vi "Process.vi"(0 "reference in":refnum<class "SSH.lvclass">, 5 "error in":errorcluster) -> (14 "reference out":refnum<class "SSH.lvclass">, 19 "error out":errorcluster)   [LabVIEW 2023, in "HPS-17000-PowerModule.lvlib" / "SSH.lvclass"]
uses:
  SSH.lvclass
  <vilib>/Utility/SystemLogging/NI_SystemLogging.lvlib
panel:
  out "error info":errorcluster
  out "Last Command":string
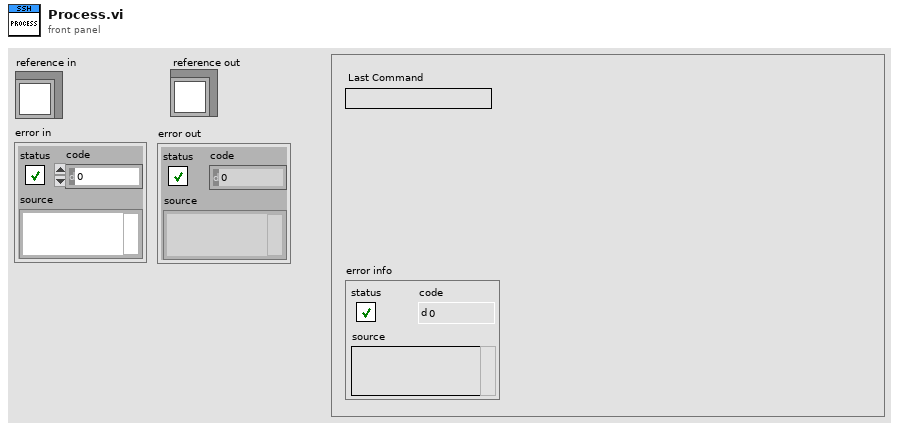
[diagram p1: front panel]
types:
  T1 = cluster{"Core":cluster{"Timeout":i32, "Events":cluster{"EventsToProcess":refnum<event-registration>}, "EventFromProcess":refnum<user-event>, "ProcessSyncQueue":refnum<queue>, "QueueFromProcess":refnum<queue>, "Command":string, "Data":variant}, "Process ID":i32, "Script Prefix":string, "Log File":string, "Full Command":string, "Script Name":string, "Standard Input":string, "Console Listbox":refnum<vi>, "Script Complete Event":refnum<user-event>}
  T2 = enum32{"Invalid", "Standard", "Closed", "Hidden", "Minimized", "Maximized"}
  T3 = cluster{"EventsToProcess":refnum<event-registration>}
  T4 = typedef "HPS-17000-PowerModule.lvlib/SSH.lvclass/ObjectAttributes.ctl" = cluster{"Update Rate (ms)":i32, "Console Listbox":refnum<vi>, "Full Command":string, "Script Name":string, "Log File":string, "IP Address":string, "Script Complete Event":refnum<user-event>}
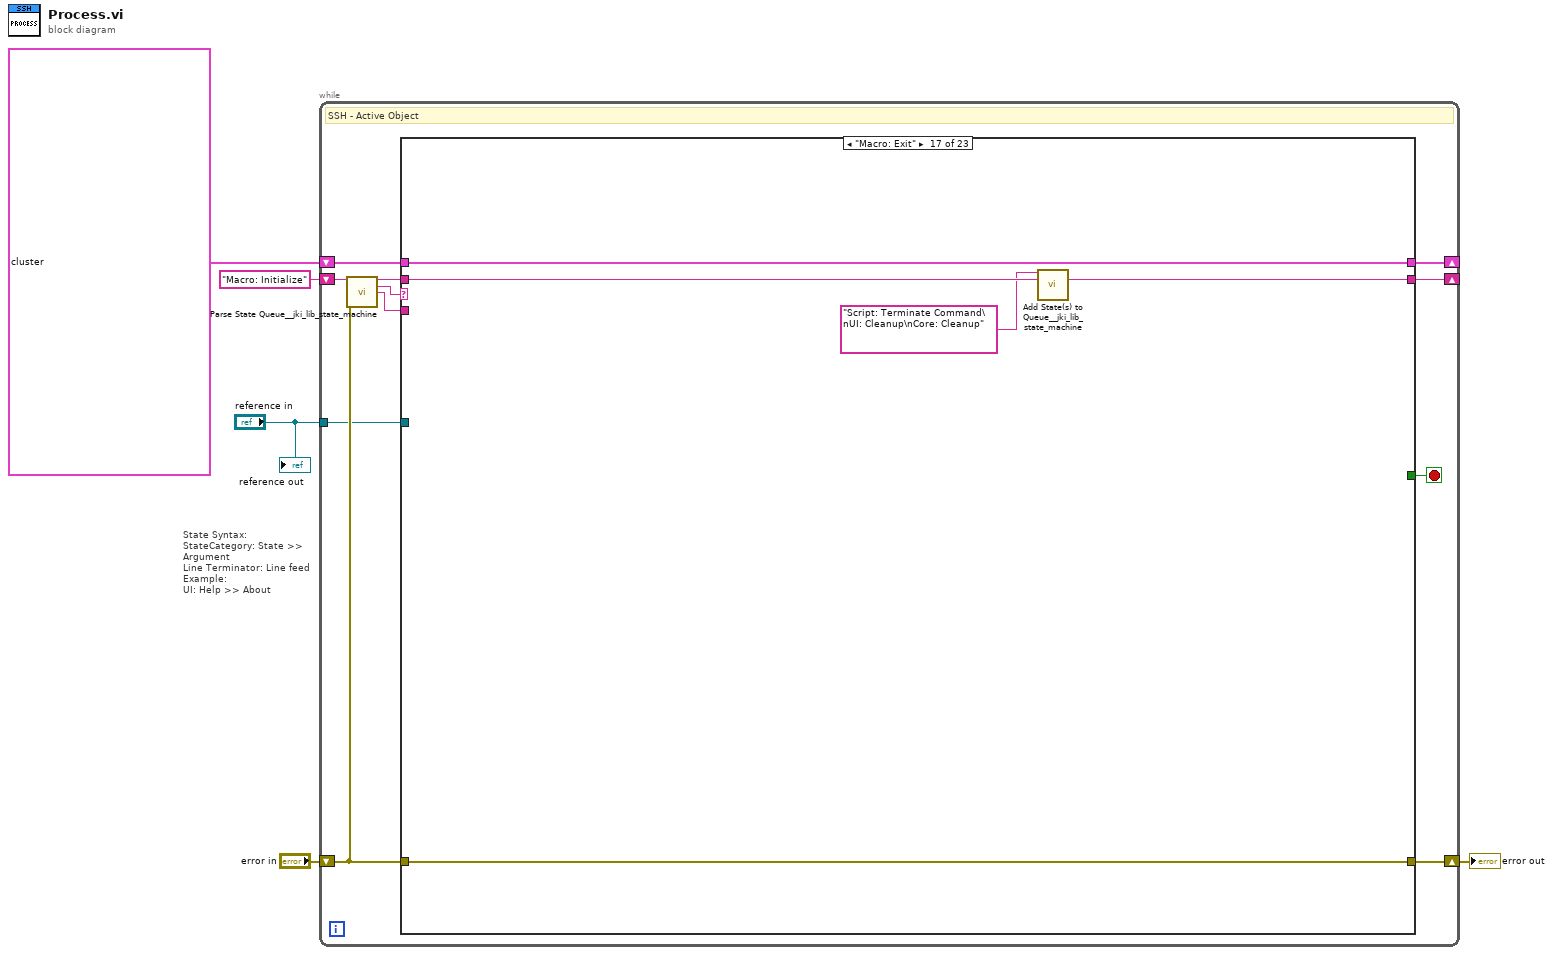
[diagram p0: block diagram]
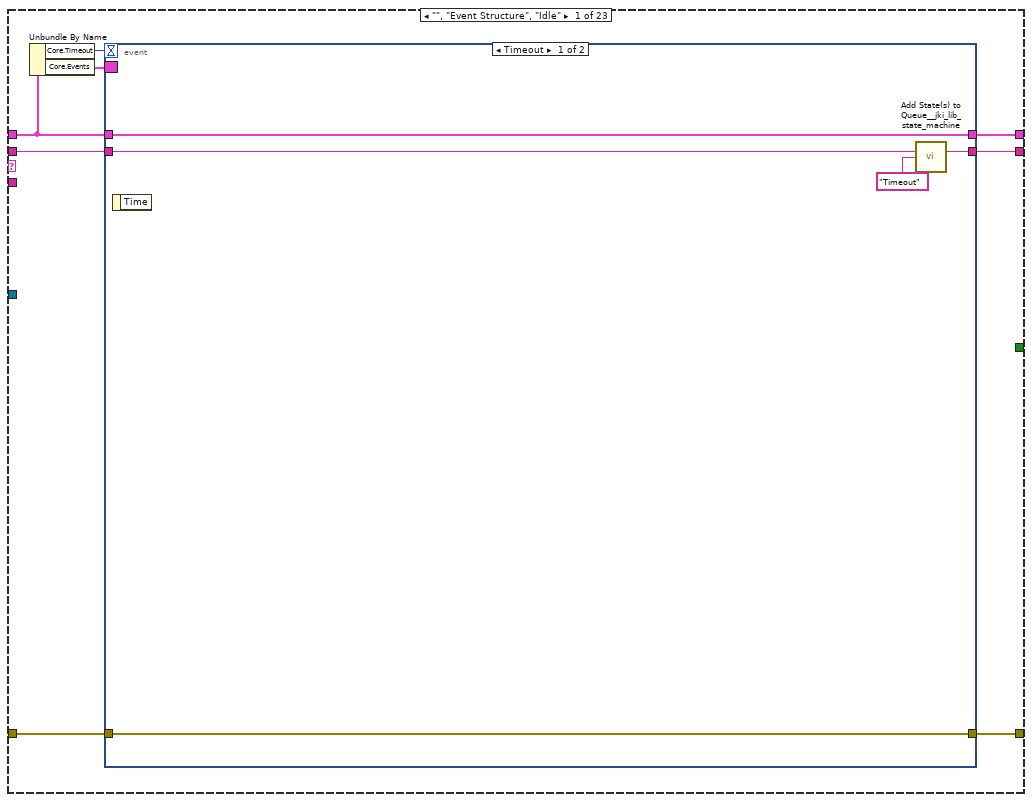
[diagram p2: hidden frame]
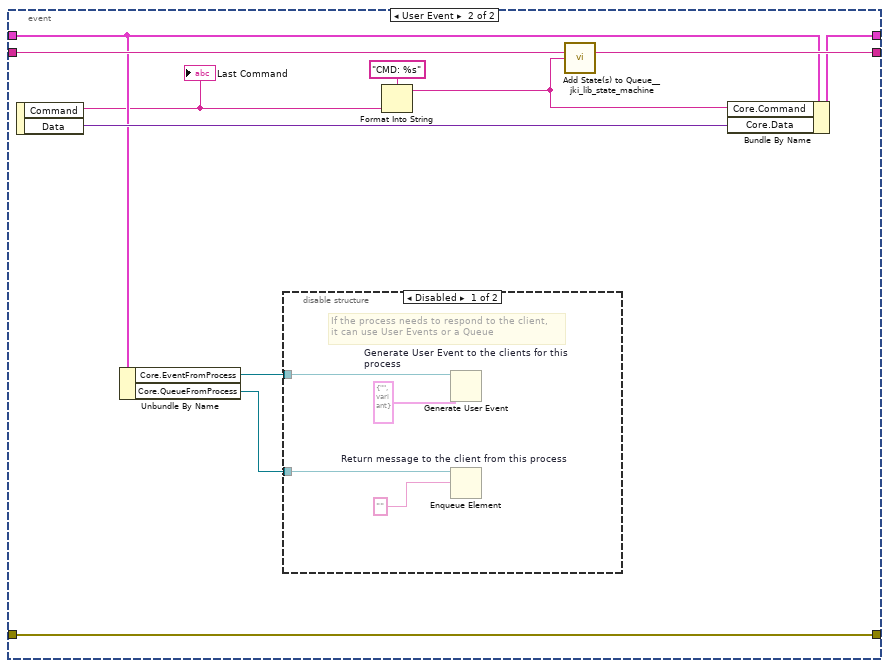
[diagram p3: hidden frame]
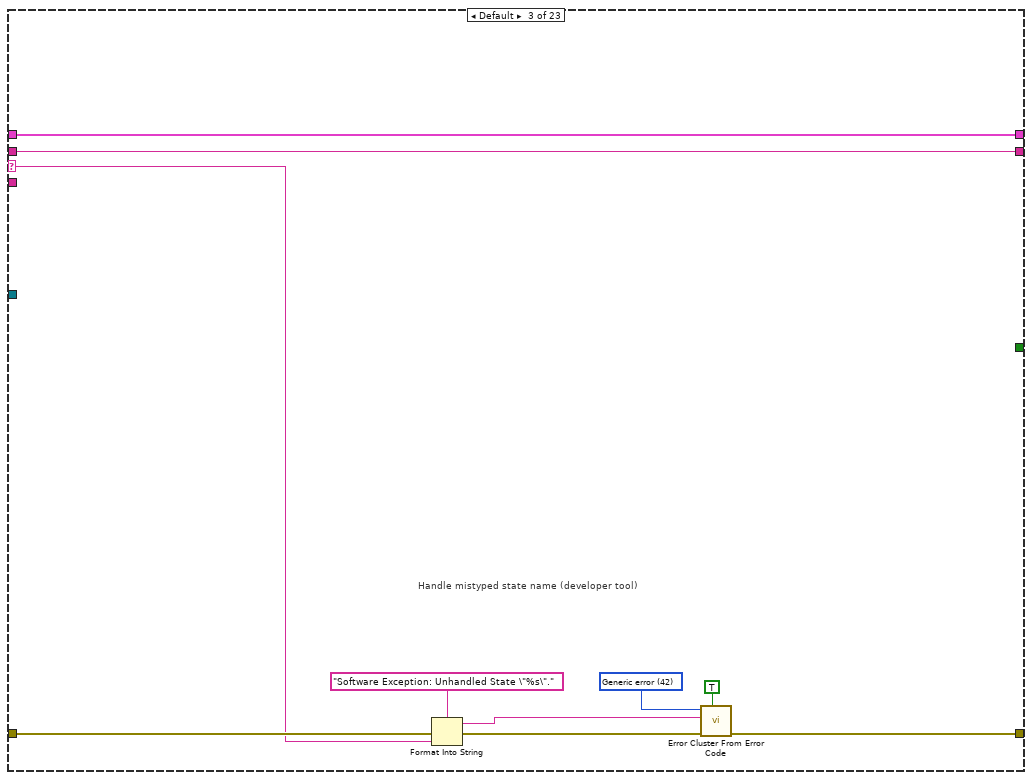
[diagram p6: hidden frame]
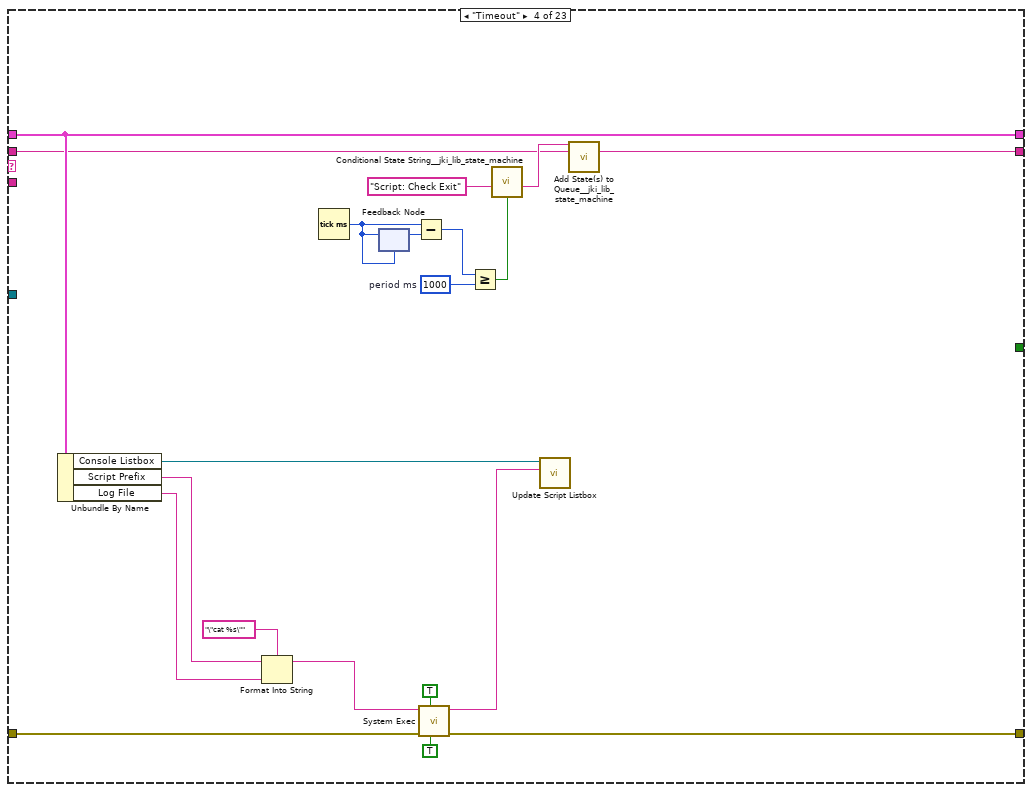
[diagram p7: hidden frame]
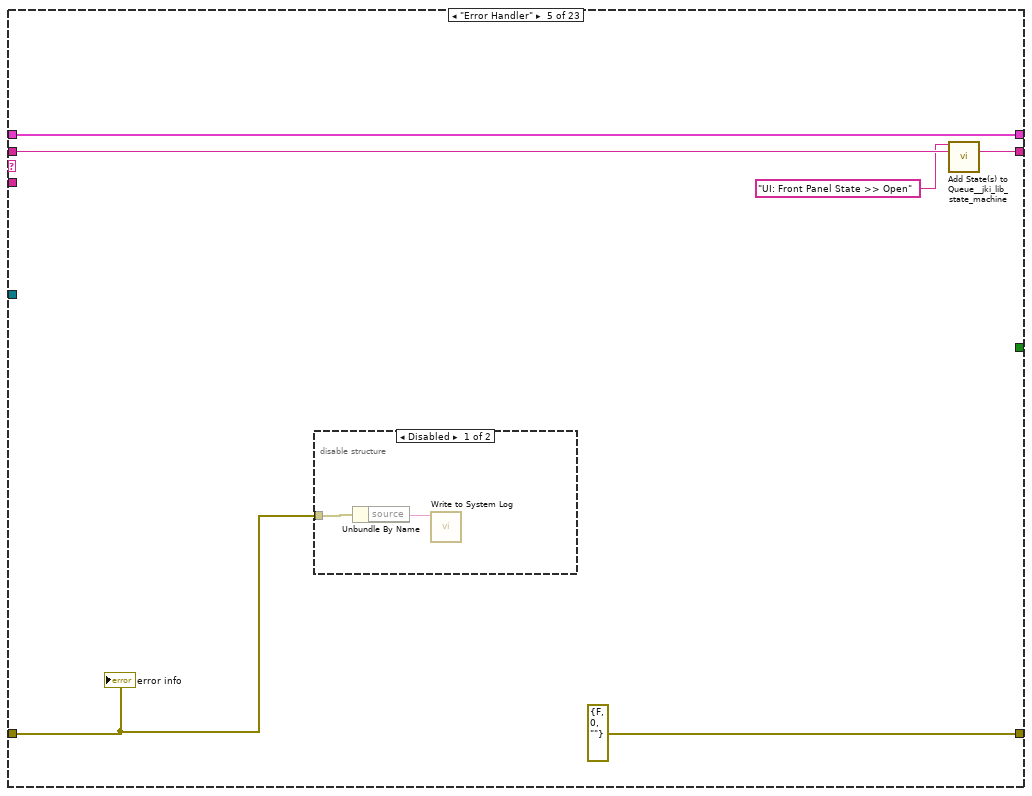
[diagram p8: hidden frame]
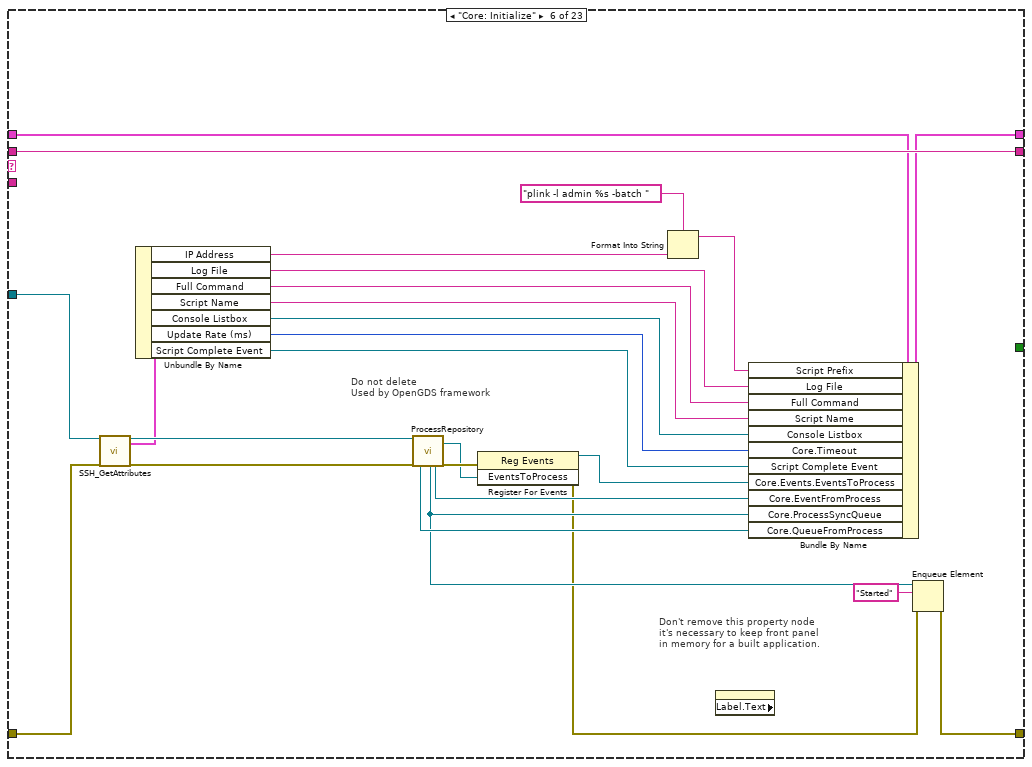
[diagram p10: hidden frame]
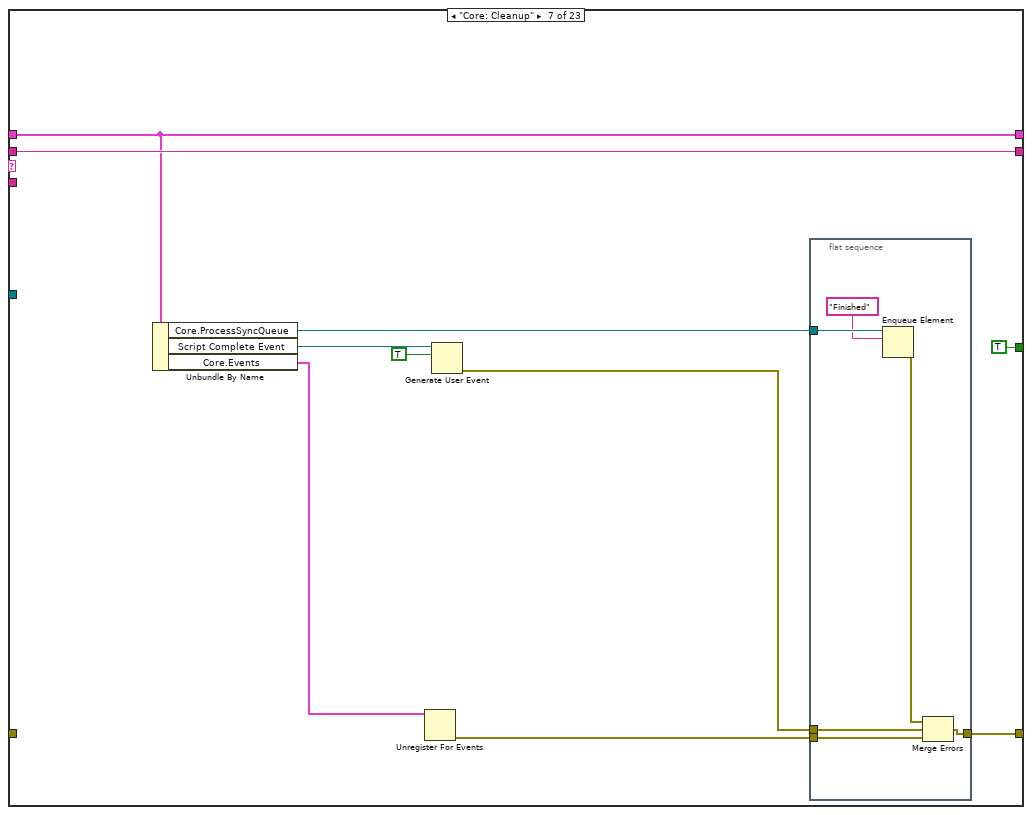
[diagram p11: hidden frame]
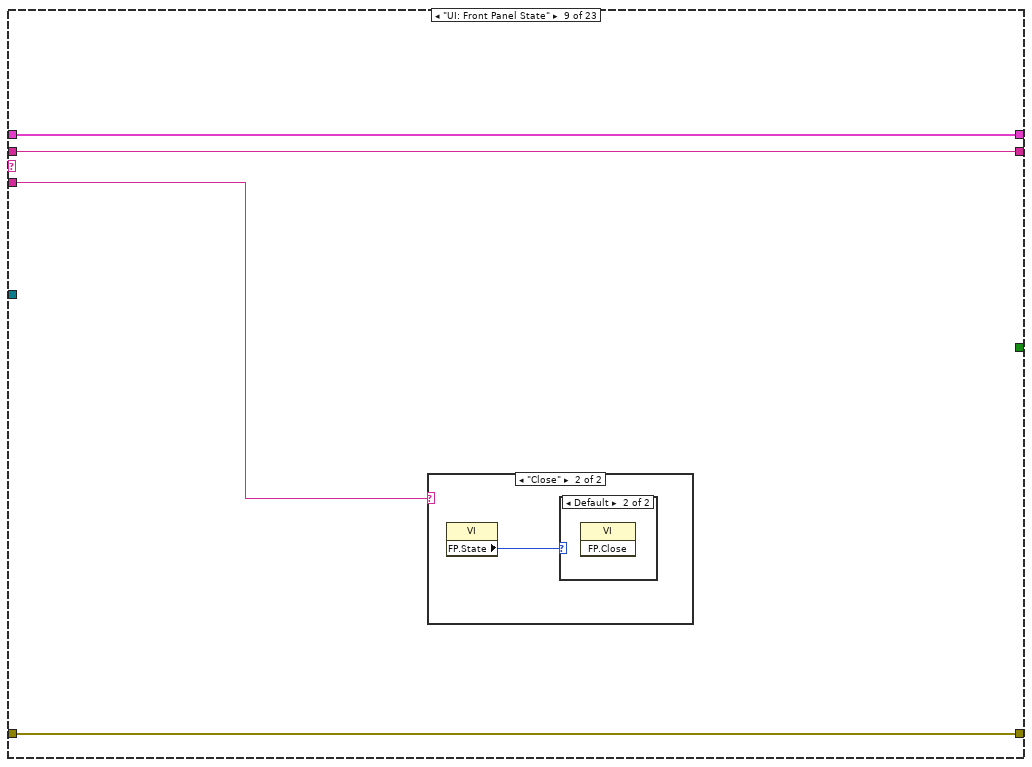
[diagram p13: hidden frame]
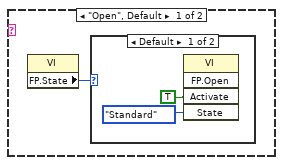
[diagram p14: hidden frame]
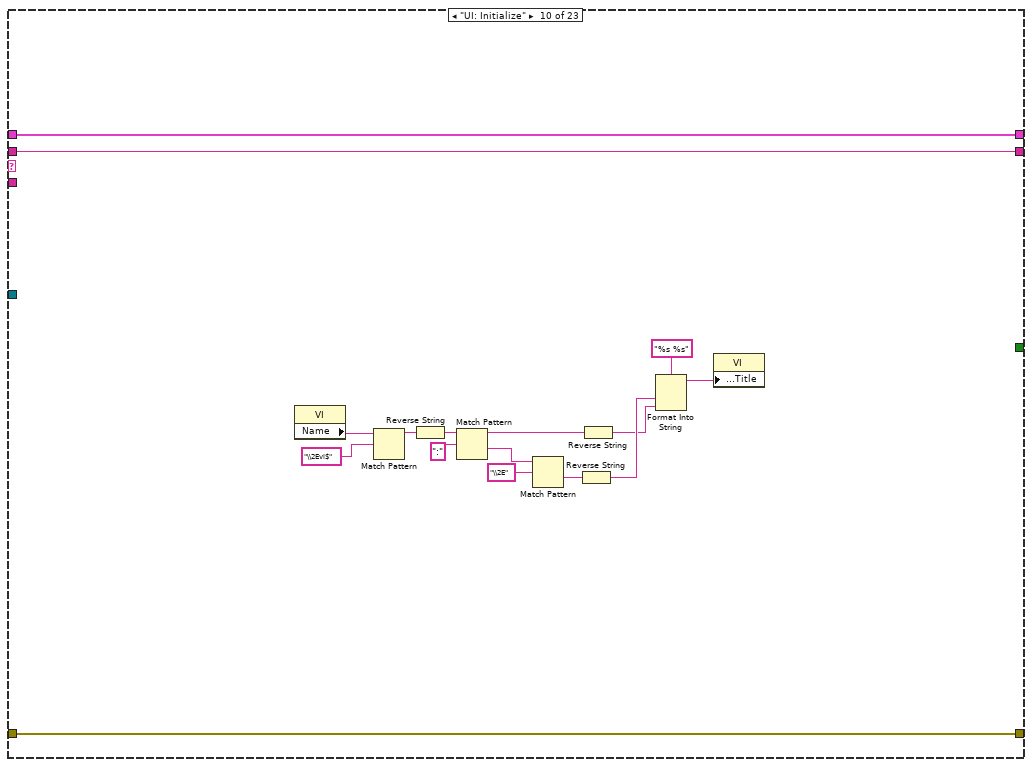
[diagram p17: hidden frame]
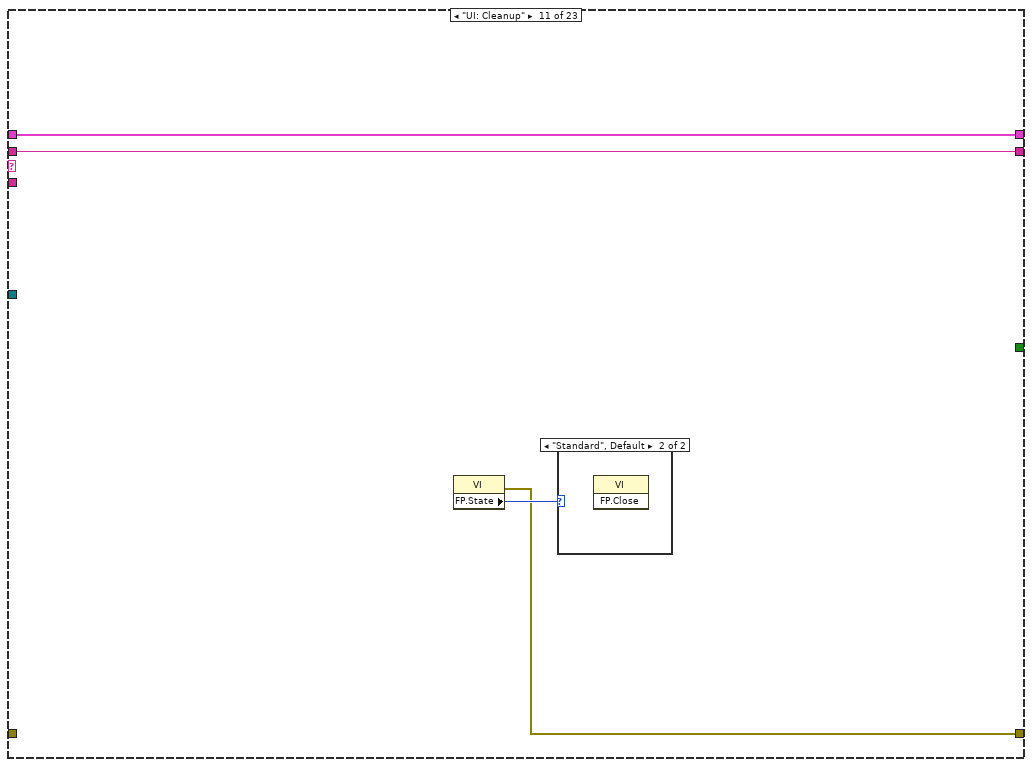
[diagram p18: hidden frame]
diagram:
  # "State Syntax:\nStateCategory: State >> Argument\nLine Terminator: Line feed\nExample:\nUI: Help >> About"
  n1 = while {
    shift-right: [w15] -> w4
    shift-left: "error in" -> [w16]
    shift-right: [w8] -> _
    shift-left: "Macro: Initialize" ("States Out") -> [w11]
    shift-right: [w14] -> _
    shift-left: T1 {"Core"={"Timeout"=-1, "Events"={"EventsToProcess"=refnum}, "EventFromProcess"=refnum, "ProcessSyncQueue"=refnum, "QueueFromProcess"=refnum, "Command"="", "Data"=variant}, "Process ID"=0, "Script Prefix"="", "Log File"="", "Full Command"="", "Script Name"="", "Standard Input"="", "Console Listbox"=refnum, "Script Complete Event"=refnum} ("LocalVariables") -> [w13]
    tunnel: "reference in" -> [w6]
    stop <- w7 stop-if-true
    # "SSH - Active Object"
    n2 = call <vilib>:"Parse State Queue__jki_lib_state_machine.vi"("State Queue"=w11, "Error In (no error)"=w16) -> ("Remaining States"=w10:string, "Current State"=w12:string, "Arguments"=w9:string)  [unwired: 11 in]
    n3 = case shown="\"Macro: Exit\"" w12 {
      selector: w12 -> [_ _ w48 _ _ _ _ _ _ _ _ _ _ _ _ _ _ _ _ _ _ _ _]
      tunnel: w16 -> [w18 w47 w50 w72 w79 w97 _ w130 w131 w154 _ w161 w164 w171 w172 w178 w183 w188 w190 w198 w218 w225 w243]
      tunnel: [w19 w47 w49 w71 errorcluster {"status"=FALSE, "code"=0, "source"=""} ("error constant") w111 w117 w130 w131 w154 w155 w161 w164 w171 w172 w178 w183 w188 w190 w197 w217 w224 w241] -> w15
      tunnel: [w24 w46 w57 w70 w83 w109 w118 w129 w133 w146 w156 w160 w163 w170 w173 w179 w184 w189 w191 w195 w214 w226 w240] -> w14
      tunnel: w13 -> [w20 w46 w57 w70 w83 w108 w118 w129 w133 w146 w156 w160 w163 w170 w173 w179 w184 w189 w191 w196 w214 w226 w240]
      tunnel: w10 -> [w22 w45 w56 w61 w82 w110 w121 w128 w134 w153 w158 w159 _ w169 w174 w177 w182 w187 w192 w205 w213 w232 w245]
      tunnel: w9 -> [_ _ _ _ _ _ _ _ w132 _ _ _ _ w166 _ _ _ _ _ _ _ _ _]
      tunnel: [w21 w45 w56 w60 w81 w110 w121 w128 w134 w153 w158 w159 "Macro: Exit" ("State(s) at Back (\"\")") w168 w174 w176 w181 w186 w192 w205 w211 w232 w245] -> w8
      tunnel: [_ _ _ _ _ _ TRUE _ _ _ _ _ _ _ _ _ _ _ _ _ _ _ _] -> w7
      tunnel: w6 -> [_ _ _ _ _ w99 _ _ _ _ _ _ _ _ _ _ _ _ _ _ _ _ _]
      frame "", "Event Structure", "Idle" {
        n4 = Unbundle By Name(w20) -> ("Core.Timeout"=w17:i32, "Core.Events"=w23:T3)
        n5 = event shown="[0] Timeout" {
          selector: w23 -> [_ _]
          dyn-events: _ -> [_ _]
          timeout: w17 -> [_ _]
          tunnel: w20 -> [w29 w33]
          tunnel: [w29 w38] -> w24
          tunnel: [w27 w40] -> w21
          tunnel: w22 -> [w28 w39]
          tunnel: [w25 w34] -> w19
          tunnel: w18 -> [w25 w34]
          event Timeout {
            n6 = event-data() -> ()  [unwired: 1 in, 1 out]
            n7 = call <vilib>:"Add State(s) to Queue__jki_lib_state_machine.vi"("State(s) in (\"\")"=w28, "State(s) at Back (\"\")"="Timeout" ("State(s) at Back (\"\")")) -> ("States Out"=w27:string)  [unwired: 13 in]
          }
          event User Event {
            n8 = event-data() -> ("Command"=w31:string, "Data"=w37:variant)  [unwired: 1 in]
            "Last Command" <- w31
            n9 = Unbundle By Name(w33) -> ("Core.EventFromProcess"=w36:refnum<user-event>, "Core.QueueFromProcess"=w35:refnum<queue>)
            n10 = disable-structure shown="Disabled" {
              disable-tunnel: w36 -> [w44 _]
              disable-tunnel: w35 -> [w43 _]
              frame Disabled {
                # "If the process needs to respond to the client,\nit can use User Events or a Queue"
                n11 = Generate User Event "Generate User Event to the clients for this process"(user event=w44, event data cluster=cluster{"Command":string, "Data":variant} {"Command"="", "Data"=variant} ("event data")) -> ()  [unwired: 2 in, 2 out]
                n12 = Enqueue Element "Return message to the client from this process"(queue=w43, element="") -> ()  [unwired: 2 in, 3 out]
              }
              frame Enabled {
              }
            }
            n13 = Format Into String(format string="CMD: %s", w31) -> (resulting string=w30:string)  [unwired: 2 in, 1 out]
            n14 = call <vilib>:"Add State(s) to Queue__jki_lib_state_machine.vi"("State(s) in (\"\")"=w39, "State(s) at Back (\"\")"=w30) -> ("States Out"=w40:string)  [unwired: 13 in]
            n15 = Bundle By Name(cluster=w33, "Core.Command"=w30, "Core.Data"=w37) -> (w38:T1)
          }
        }
      }
      frame "---------- Core ----------" {
      }
      frame Default {
        w54 = 42 items=["No error", "Argument error", "Memory is full", "Out of zone", "End of file", "File already open", "Generic file I/O error", "File not found", "File permission error", "Disk is full", "Duplicate path", "Too many files open", "System feature not enabled", "Resource file not found", "Cannot add resource", "Resource not found", "Image not found", "Image memory error", "Pen does not exist", "Config type invalid", "Config token not found", "Config parse error", "Config memory error", "Bad external code format", "Bad external code offset", "External code not present", "Null window", "Destroy window error", "Null menu", "Print aborted", "Bad print record", "Print driver error", "Windows error during printing", "Memory error during printing", "Print dialog error", "Generic print error", "Invalid device refnum", "Device not found", "Device parameter error", "Device unit error", "Cannot open device", "Device call aborted", "Generic error", "Cancelled by user", "Object ID too low", "Object ID too high", "Object not in heap", "Unknown heap", "Unknown object (invalid DefProc)", "Unknown object (DefProc not in table)", "Message out of range", "Invalid (null) method", "Unknown message", "Manager call not supported", "Bad address", "Network operation in progress", "Network operation timed out", "Connection is busy", "Network attribute not supported", "Network error", "Address in use", "System out of memory", "Connection aborted", "Connection refused", "Not connected", "Already connected", "Connection closed", "Initialization error (interapplication manager)", "Bad occurrence", "Wait on unbound occurrence handler", "Occurrence queue overflow", "Datalog type conflict", "Unused", "Unrecognized type (interapplication manager)", "Memory corrupt", "Failed to make temporary DLL", "Old CIN version", "Drag socket not found", "Failed to load drop-object", "Failed to register OLE object", "Failed to release OLE object", "Format specifier type mismatch", "Unknown format specifier", "Too few format specifiers", "Too many format specifiers", "Scan failed", "Newer CIN version", "Error converting to variant", "Runtime menu error", "Password tampered", "Variant attribute not found", "Incompatible variant data type", "Event data is not available", "Event Store is not present", "Occurrence is not found", "Event Queue is not created", "Event info is not available", "Refnum passed is NULL", "Error retrieving Class GUID", "Error retrieving CoClass GUID", "Error retrieving TypeLib GUID.", "Bad built application magic bytes.", "Specific driver is different from the specific driver associated with the Logical Name.", "There is no session opened to the class driver.", "Max Error", "MAX - Error with config objects", "MAX - Error loading configuration", "MAX - Group not supported"]
        # "Handle mistyped state name (developer tool)"
        n16 = Format Into String(format string="Software Exception: Unhandled State \"%s\"." ("message"), error in=w50, w48) -> (resulting string=w53:string, error out=w52:errorcluster)  [unwired: 1 in]
        n17 = call <vilib>:"Error Cluster From Error Code.vi"("show call chain? (False)"=TRUE, "error in (no error)"=w52, "error message (\"\")"=w53, "error code (0)"=w54) -> ("error out"=w49:errorcluster)  [unwired: 5 in]
      }
      frame "Timeout" {
        w66 = u32 1000  # period ms
        n18 = Unbundle By Name(w70) -> ("Console Listbox"=w69:refnum<vi>, "Script Prefix"=w67:string, "Log File"=w68:string)
        n19 = Format Into String(format string="\"cat %s\"", initial string=w67, w68) -> (resulting string=w74:string)  [unwired: 1 in, 1 out]
        n20 = Tick Count (ms)() -> (millisecond timer value=w58:u32)
        n21 = feedback-in #1(w58) -> ()
        n22 = feedback #1(w58) -> (w59:u32)
        n23 = Subtract(x=w58, y=w59) -> (x-y=w64:u32)
        n24 = call <vilib>:"System Exec.vi"("run minimized? (F)"=TRUE, "wait until completion? (T)"=TRUE, "error in (no error)"=w72, "command line"=w74) -> ("error out"=w71:errorcluster, "standard output"=w73:string)  [unwired: 4 in, 2 out]
        n25 = Greater Or Equal?(x=w64, y=w66) -> (x >= y?=w65:bool)
        n26 = call <vilib>:"Conditional State String__jki_lib_state_machine.vi"("Do State(s)?"=w65, "State"="Script: Check Exit") -> ("State Out"=w63:string)  [unwired: 7 in]
        n27 = call "Update Script Listbox.vi"("standard output"=w73, "ListBox in"=w69) -> ()  [unwired: 10 in]
        n28 = call <vilib>:"Add State(s) to Queue__jki_lib_state_machine.vi"("State(s) in Front (\"\")"=w63, "State(s) in (\"\")"=w61) -> ("States Out"=w60:string)  [unwired: 13 in]
      }
      frame "Error Handler" {
        n29 = disable-structure shown="Disabled" {
          disable-tunnel: w79 -> [w85 _]
          frame Disabled {
            n30 = Unbundle By Name(w85) -> ("source"=w84:string)
            n31 = call <vilib>:"Write to System Log.vi"("message"=w84) -> ()  [unwired: 10 in, 1 out]
          }
          frame Enabled {
          }
        }
        n32 = call <vilib>:"Add State(s) to Queue__jki_lib_state_machine.vi"("State(s) in Front (\"\")"="UI: Front Panel State >> Open" ("State(s) at Back (\"\")"), "State(s) in (\"\")"=w82) -> ("States Out"=w81:string)  [unwired: 13 in]
        "error info" <- w79
      }
      frame "Core: Initialize" {
        # "Do not delete\nUsed by OpenGDS framework"
        # "Don't remove this property node\nit's necessary to keep front panel\nin memory for a built application."
        # "Template created by VI Technologies"
        n33 = call "SSH_GetAttributes.vi"("reference in"=w99, "Error In"=w97) -> ("reference out"=w98:refnum<class "SSH.lvclass">, "Data"=w94:T4, "Error Out"=w96:errorcluster)  [unwired: 14 in, 1 out]
        n34 = Unbundle By Name(w94) -> ("IP Address"=w93:string, "Log File"=w86:string, "Full Command"=w92:string, "Script Name"=w91:string, "Console Listbox"=w89:refnum<vi>, "Update Rate (ms)"=w90:i32, "Script Complete Event"=w88:refnum<user-event>)
        n35 = call "ProcessRepository.vi"("reference in"=w98, "Error In"=w96) -> ("QueueFromProcess"=w103:refnum<queue>, "ProcessSyncQueue"=w101:refnum<queue>, "EventFromProcess"=w104:refnum<user-event>, "EventsToProcess"=w106:refnum<user-event>, "Error Out"=w107:errorcluster)  [unwired: 10 in, 3 out]
        n36 = register-events(error in=w107, w106) -> (reference out=w105:refnum<event-registration>, error out=w100:errorcluster)  [unwired: 1 in]
        n37 = Format Into String(format string="plink -l admin %s -batch ", w93) -> (resulting string=w87:string)  [unwired: 2 in, 1 out]
        n38 = property on="reference in" class="LVClassControl (strict)" props=["Label", "Text"]() -> ()  [unwired: 2 in, 3 out]
        n39 = Bundle By Name(cluster=w108, "Script Prefix"=w87, "Log File"=w86, "Full Command"=w92, "Script Name"=w91, "Console Listbox"=w89, "Core.Timeout"=w90, "Script Complete Event"=w88, "Core.Events.EventsToProcess"=w105, "Core.EventFromProcess"=w104, "Core.ProcessSyncQueue"=w101, "Core.QueueFromProcess"=w103) -> (w109:T1)
        n40 = Enqueue Element(queue=w101, element="Started", error in (no error)=w100) -> (error out=w111:errorcluster)  [unwired: 1 in, 2 out]
      }
      frame "Core: Cleanup" {
        n41 = Unbundle By Name(w118) -> ("Core.ProcessSyncQueue"=w119:refnum<queue>, "Script Complete Event"=w114:refnum<user-event>, "Core.Events"=w115:T3)
        n42 = Unregister For Events(event registration refnum=w115) -> (error out=w116:errorcluster)  [unwired: 1 in]
        n43 = Generate User Event(user event=w114, event data cluster=TRUE ("event data")) -> (error out=w112:errorcluster)  [unwired: 2 in, 1 out]
        n44 = flat-sequence {
          tunnel: [w127] -> w117
          tunnel: w119 -> [w126]
          tunnel: w116 -> [w125]
          tunnel: w112 -> [w122]
          frame #0 {
            n45 = Enqueue Element(queue=w126, element="Finished") -> (error out=w123:errorcluster)  [unwired: 2 in, 2 out]
            n46 = Merge Errors(w123, w122, w125) -> (w127:errorcluster)
          }
        }
      }
      frame "---------- UI ----------" {
      }
      frame "UI: Front Panel State" {
        n47 = case shown="\"Close\"" w132 {
          frame "Open", Default {
            n48 = property class="VI"() -> ("FP.State"=w135:T2)  [unwired: 2 in, 2 out]
            n49 = case shown="Default" w135 {
              frame Default {
                n50 = invoke class="VI" method="FP.Open"("Activate"=TRUE, "State"=T2."Standard") -> ()  [unwired: 3 in, 5 out]
              }
              frame "Standard" {
              }
            }
          }
          frame "Close" {
            n51 = property class="VI"() -> ("FP.State"=w138:T2)  [unwired: 2 in, 2 out]
            n52 = case shown="Default" w138 {
              frame "Closed" {
              }
              frame Default {
                n53 = invoke class="VI" method="FP.Close"() -> ()  [unwired: 3 in, 3 out]
              }
            }
          }
        }
      }
      frame "UI: Initialize" {
        n54 = property class="VI"() -> ("Name"=w152:string)  [unwired: 2 in, 2 out]
        n55 = Match Pattern(string=w152, regular expression="\\2Evi$") -> (before substring=w150:string)  [unwired: 1 in, 3 out]
        n56 = Reverse String(1:w150) -> (0:w149:string)
        n57 = Match Pattern(string=w149, regular expression=":") -> (before substring=w147:string, after substring=w145:string)  [unwired: 1 in, 2 out]
        n58 = Match Pattern(string=w145, regular expression="\\2E") -> (after substring=w143:string)  [unwired: 1 in, 3 out]
        n59 = Reverse String(1:w143) -> (0:w142:string)
        n60 = Reverse String(1:w147) -> (0:w141:string)
        n61 = Format Into String(format string="%s %s", w142, w141) -> (resulting string=w140:string)  [unwired: 2 in, 1 out]
        n62 = property class="VI"("Front Panel.Title"=w140) -> ()  [unwired: 2 in, 2 out]
      }
      frame "UI: Cleanup" {
        n63 = property class="VI"() -> (error out=w155:errorcluster, "FP.State"=w157:T2)  [unwired: 2 in, 1 out]
        n64 = case shown="\"Standard\", Default" w157 {
          frame "Closed" {
          }
          frame "Standard", Default {
            n65 = invoke class="VI" method="FP.Close"() -> ()  [unwired: 3 in, 3 out]
          }
        }
      }
      frame "---------- CMD ----------" {
      }
      frame "CMD: Exit" {
      }
      frame "CMD: Front Panel State" {
        n66 = Format Into String(format string="UI: Front Panel State>>%s" ("string"), w166) -> (resulting string=w165:string)  [unwired: 2 in, 1 out]
        n67 = call <vilib>:"Add State(s) to Queue__jki_lib_state_machine.vi"("State(s) in (\"\")"=w169, "State(s) at Back (\"\")"=w165) -> ("States Out"=w168:string)  [unwired: 13 in]
      }
      frame "---------- Macro ----------" {
      }
      frame "Macro: Initialize" {
        n68 = call <vilib>:"Add State(s) to Queue__jki_lib_state_machine.vi"("State(s) in Front (\"\")"="Core: Initialize\nUI: Initialize\nScript: Check Running\nScript: Run Command\nScript: Check Running" ("States Out"), "State(s) in (\"\")"=w177) -> ("States Out"=w176:string)  [unwired: 13 in]
      }
      frame "Macro: Exit" {
        n69 = call <vilib>:"Add State(s) to Queue__jki_lib_state_machine.vi"("State(s) in Front (\"\")"="Script: Terminate Command\nUI: Cleanup\nCore: Cleanup", "State(s) in (\"\")"=w182) -> ("States Out"=w181:string)  [unwired: 13 in]
      }
      frame "Macro: Script Complete" {
        n70 = call <vilib>:"Add State(s) to Queue__jki_lib_state_machine.vi"("State(s) in Front (\"\")"="UI: Cleanup\nCore: Cleanup", "State(s) in (\"\")"=w187) -> ("States Out"=w186:string)  [unwired: 13 in]
      }
      frame "---------- Script ----------" {
      }
      frame "Script: Check Running" {
        n71 = Unbundle By Name(w196) -> ("Script Prefix"=w193:string, "Script Name"=w194:string)
        n72 = Format Into String(format string="\"pgrep %s\"", initial string=w193, w194) -> (resulting string=w201:string)  [unwired: 1 in, 1 out]
        n73 = call <vilib>:"System Exec.vi"("run minimized? (F)"=TRUE, "wait until completion? (T)"=TRUE, "error in (no error)"=w198, "command line"=w201) -> ("error out"=w197:errorcluster, "standard output"=w200:string)  [unwired: 4 in, 2 out]
        n74 = Decimal String To Number(string=w200) -> (number=w199:i32)  [unwired: 2 in, 1 out]
        n75 = Bundle By Name(cluster=w196, "Process ID"=w199) -> (w195:T1)
      }
      frame "Script: Check Exit" {
        n76 = Unbundle By Name(w214) -> ("Script Prefix"=w215:string, "Script Name"=w216:string)
        n77 = Format Into String(format string="\"pgrep %s\"", initial string=w215, w216) -> (resulting string=w219:string)  [unwired: 1 in, 1 out]
        n78 = call <vilib>:"System Exec.vi"("run minimized? (F)"=TRUE, "wait until completion? (T)"=TRUE, "error in (no error)"=w218, "command line"=w219) -> ("error out"=w217:errorcluster, "standard output"=w210:string)  [unwired: 4 in, 2 out]
        n79 = Decimal String To Number(string=w210) -> (number=w208:i32)  [unwired: 2 in, 1 out]
        n80 = Greater Than 0?(x=w208) -> (x > 0?=w207:bool)
        n81 = Not(x=w207) -> (.not. x?=w206:bool)
        n82 = call <vilib>:"Conditional State String__jki_lib_state_machine.vi"("Do State(s)?"=w206, "State"="Macro: Script Complete") -> ("State Out"=w212:string)  [unwired: 7 in]
        n83 = call <vilib>:"Add State(s) to Queue__jki_lib_state_machine.vi"("State(s) in Front (\"\")"=w212, "State(s) in (\"\")"=w213) -> ("States Out"=w211:string)  [unwired: 13 in]
      }
      frame "Script: Run Command" {
        n84 = Unbundle By Name(w226) -> ("Process ID"=w231:i32, "Script Prefix"=w227:string, "Full Command"=w228:string, "Standard Input"=w223:string)
        n85 = Format Into String(format string="\"%s\"", initial string=w227, w228) -> (resulting string=w229:string)  [unwired: 1 in, 1 out]
        n86 = case shown="0" w231 {
          tunnel: w225 -> [w233 w237]
          tunnel: [w233 w236] -> w224
          tunnel: w229 -> [_ w235]
          tunnel: w223 -> [_ w234]
          frame Default {
            # "process already running\ndont launch again"
          }
          frame 0 {
            # "process not running\nlaunch it"
            n87 = call <vilib>:"System Exec.vi"("run minimized? (F)"=TRUE, "wait until completion? (T)"=FALSE, "error in (no error)"=w237, "standard input"=w234, "command line"=w235) -> ("error out"=w236:errorcluster)  [unwired: 3 in, 3 out]
          }
        }
      }
      frame "Script: Terminate Command" {
        n88 = Unbundle By Name(w240) -> ("Script Prefix"=w242:string, "Process ID"=w244:i32)
        n89 = case shown="Default" w244 {
          selector: w244 -> [w248 _]
          tunnel: w243 -> [w251 w254]
          tunnel: [w250 w254] -> w241
          tunnel: w242 -> [w246 _]
          frame Default {
            n90 = Format Into String(format string="\"kill %d\"", initial string=w246, w248) -> (resulting string=w247:string)  [unwired: 1 in, 1 out]
            n91 = call <vilib>:"System Exec.vi"("run minimized? (F)"=TRUE, "wait until completion? (T)"=TRUE, "error in (no error)"=w251, "command line"=w247) -> ("error out"=w250:errorcluster)  [unwired: 4 in, 3 out]
          }
          frame 0 {
            # "process not running\nnothing to terminate"
          }
        }
      }
    }
  }
  "error out" <- w4
  "reference out" <- "reference in"
